vi "Read Cal Coefficients File.vi"() -> (0 "Original Coefficients":T1[](array[typedef]) {"Elapsed Time" format="%<%H:%M:%S>t"; "zero_utc" format="%x"; "cal_utc" format="%x"; "Pump Flow Rate" format="%0d"; "Number of Zeroes" format="%0d"; "V2C" format="%0d"; "C2V" format="%0d"; "duration" format="%<%H:%M:%S>t"; "DAC" format="%03x"; "mI" format="%.3g"; "V_(RA,15mA)" format="%0.4f"; "V_(RA,5mA)" format="%0.4f"; "Chamber Temp" format="%.1f"; "Humidity" format="%.1f"}, 1 "DATE":string, 2 "TYPE":string, 3 "CalFile Selected":path, 4 "PCB":string, 5 "Error":bool)   [LabVIEW 2016]
uses:
  Controls/Calibration Coefficients.ctl
  <vilib>/regexp/Match Regular Expression.xnode
panel:
  out "Lowc2v index":i32
  out "LowC2V":sgl[][](array[numeric]) format="%.3g"
  out "Lowc2v:size":i32
  out "End":bool
  out "Channel":string
  out "v2c index":i32
  out "c2v index":u8
  out "Char_current":sgl
  out "v2c:size":i32
  out "c2v:size":i32
  out "V2C":sgl[][](array[numeric]) format="%.3g"
  out "Spreadsheet":string[][](array[string])
  out "C2V":sgl[][](array[numeric]) format="%.3g"
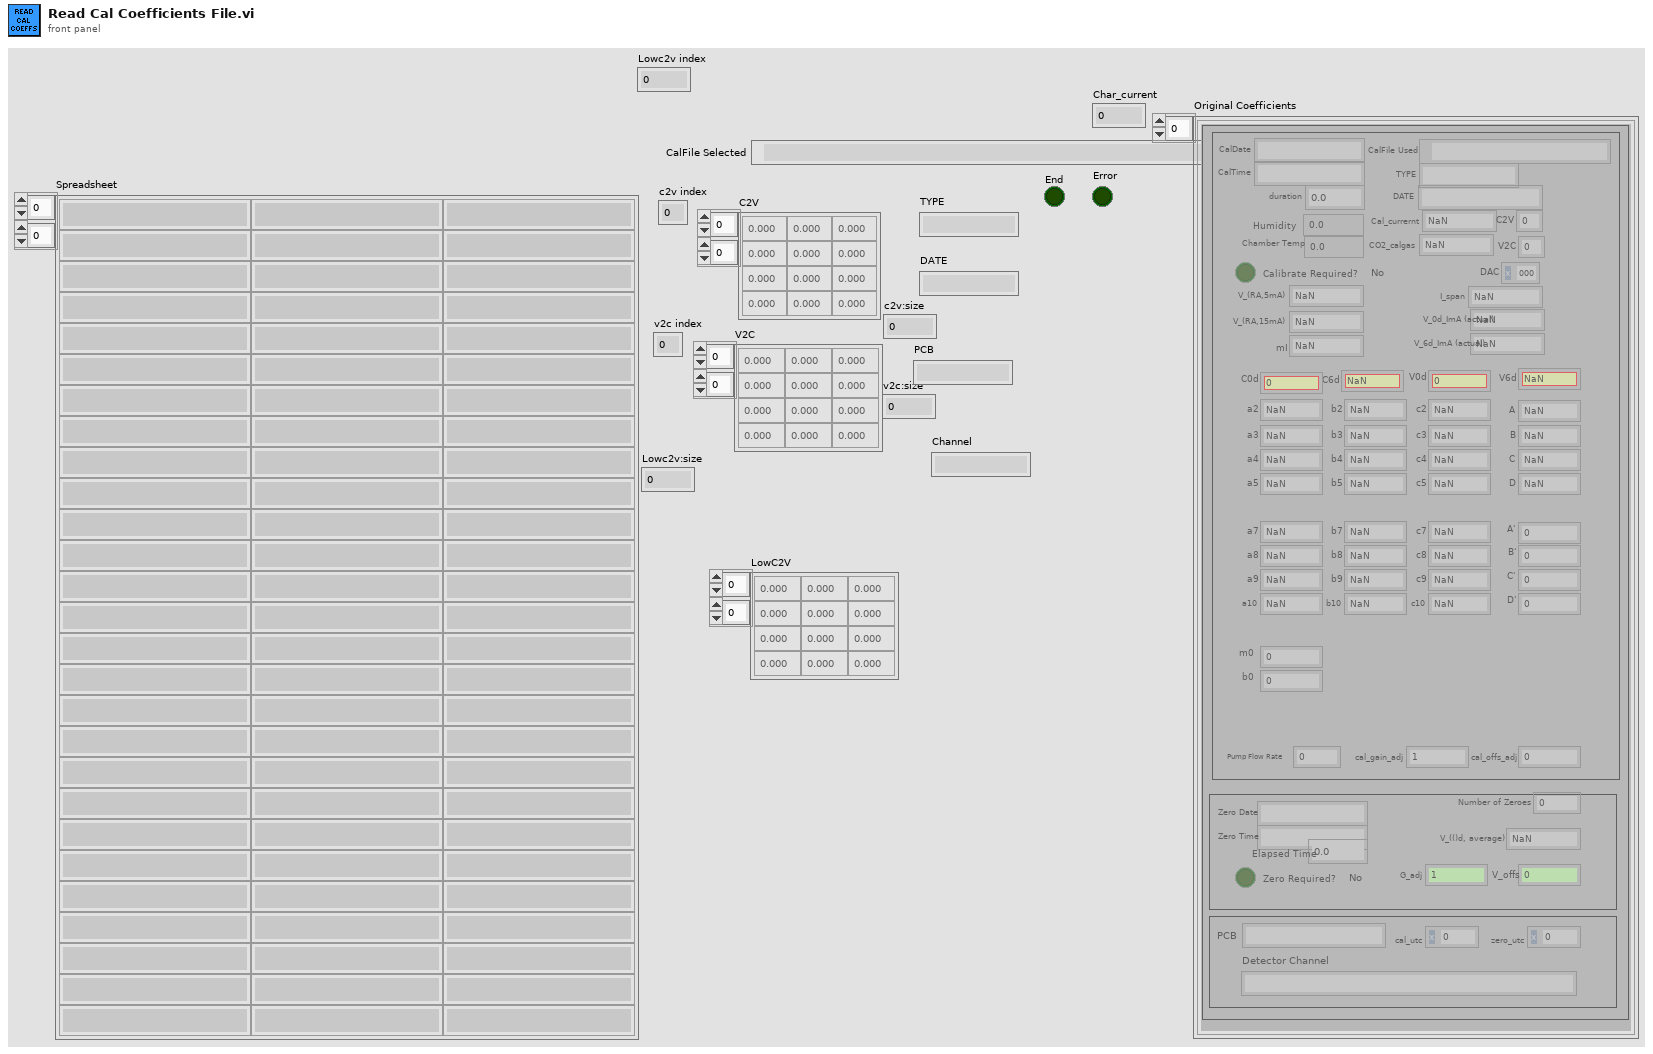
[diagram p1: front panel]
types:
  T1 = typedef "Calibration Coefficients.ctl" = cluster{"CalFile Used":path, "TYPE":string, "DATE":string, "Humidity":sgl, "Chamber Temp":dbl, "CO2_calgas":dbl, "V_(RA,5mA)":dbl, "V_(RA,15mA)":dbl, "mI":dbl, "V_0d_ImA (actual)":dbl, "V_6d_ImA (actual)":dbl, "I_span":dbl, "DAC":u16, "A":dbl, "B":dbl, "C":dbl, "D":dbl, "V6d":dbl, "A'":dbl, "B'":dbl, "C'":dbl, "D'":dbl, "V0d":dbl, "CalDate":string, "CalTime":string, "duration":dbl, "Detector Channel":string, "a2":dbl, "a3":dbl, "a4":dbl, "a5":dbl, "b2":dbl, "c2":dbl, "b3":dbl, "c3":dbl, "b4":dbl, "c4":dbl, "b5":dbl, "c5":dbl, "a7":dbl, "a8":dbl, "a9":dbl, "a10":dbl, "b7":dbl, "b8":dbl, "b9":dbl, "b10":dbl, "c7":dbl, "c8":dbl, "c9":dbl, "c10":dbl, "cal_offs_adj":dbl, "cal_gain_adj":dbl, "C6d":dbl, "C0d":dbl, "Cal_currernt":dbl, "C2V":u16, "V2C":u16, "Zero Date":string, "Zero Time":string, "Number of Zeroes":u16, "V_(()d, average)":dbl, "V_offs ":dbl, "G_adj":dbl, "Pump Flow Rate":u16, "Zero Required? ":bool, "Calibrate Required?":bool, "cal_utc":dbl, "zero_utc":dbl, "Elapsed Time":dbl, "PCB":string, "m0":dbl, "b0":dbl}
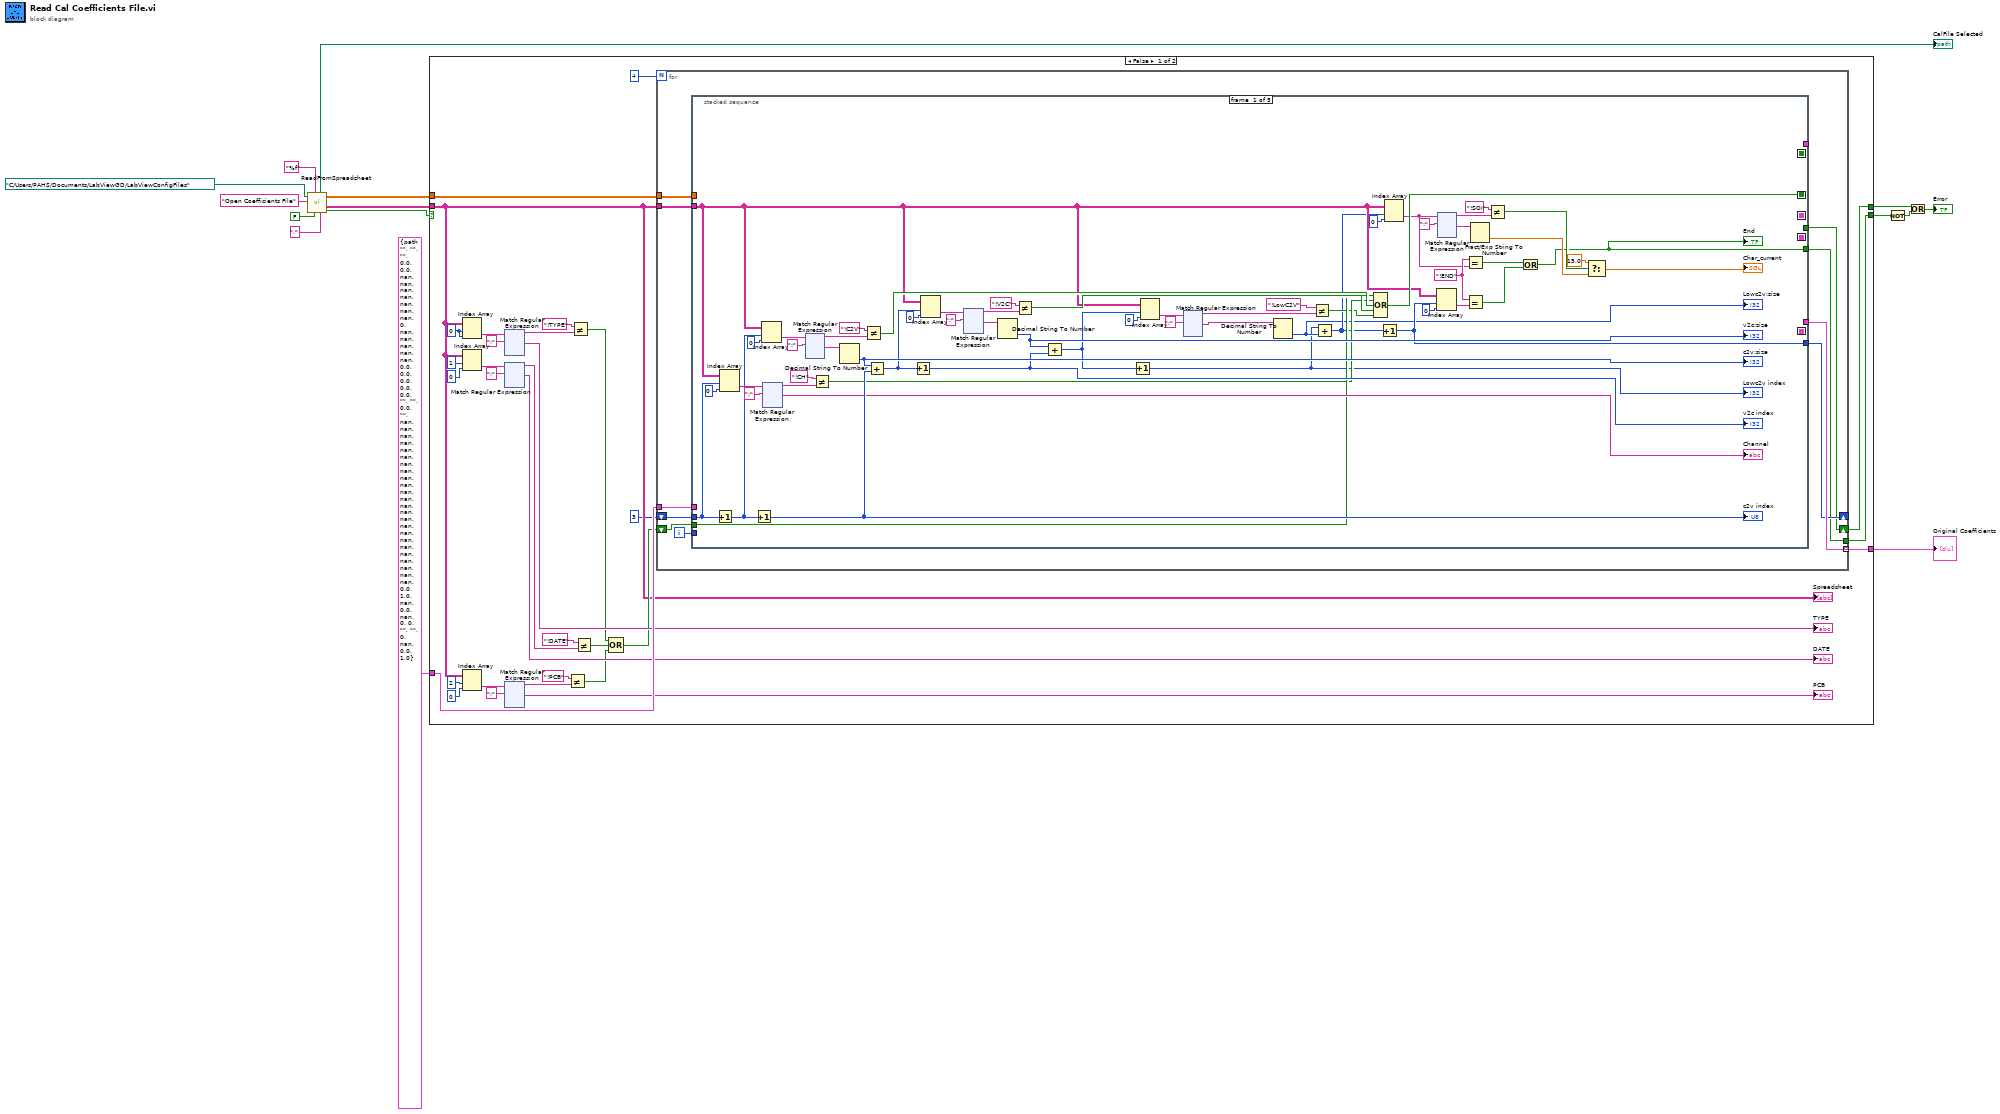
[diagram p0: block diagram]
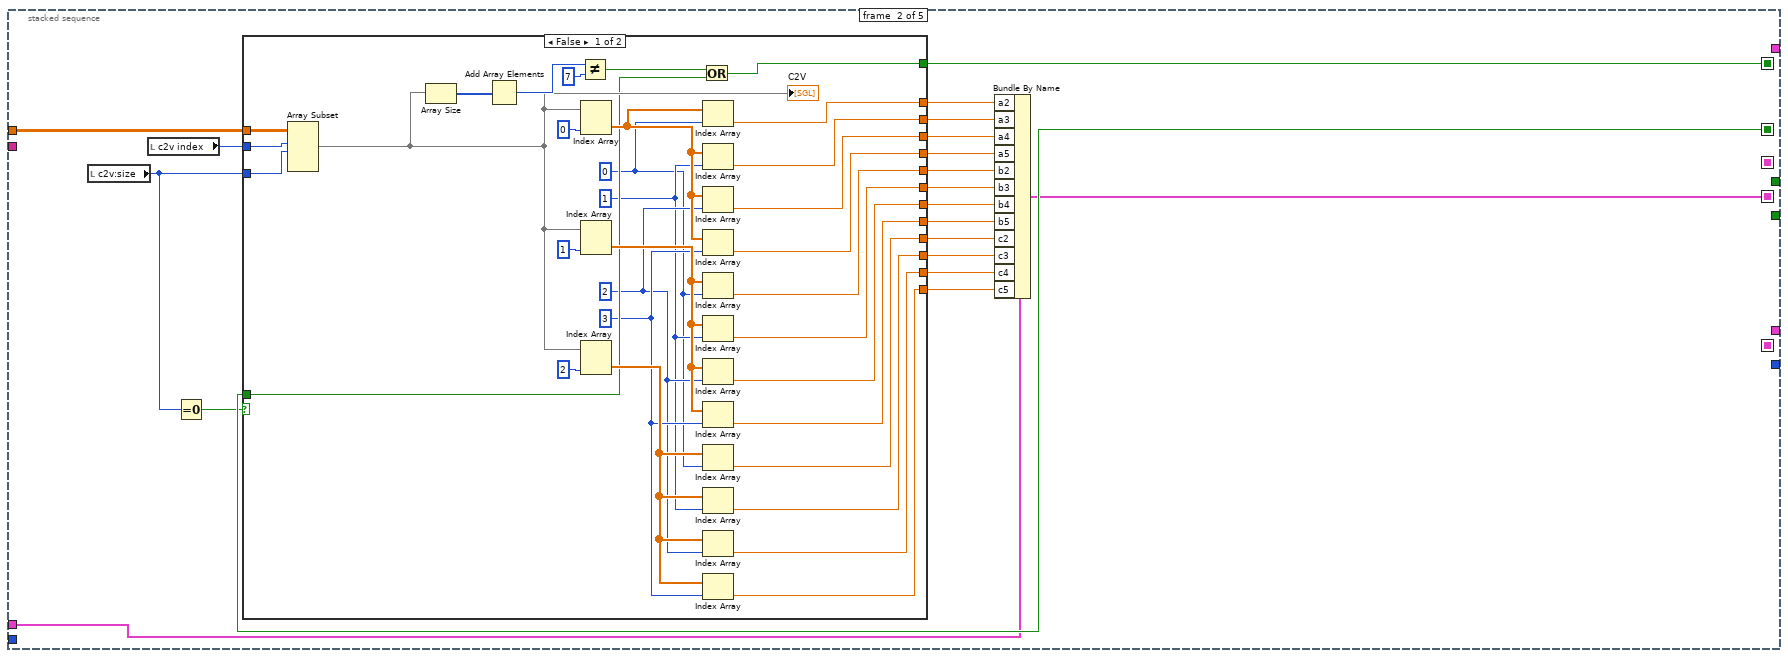
[diagram p2: hidden frame]
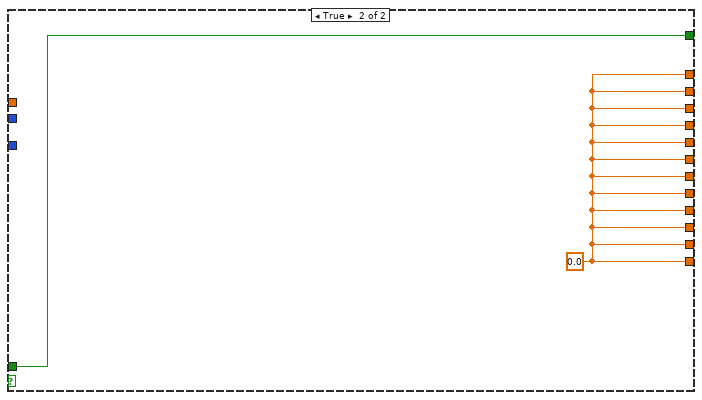
[diagram p3: hidden frame]
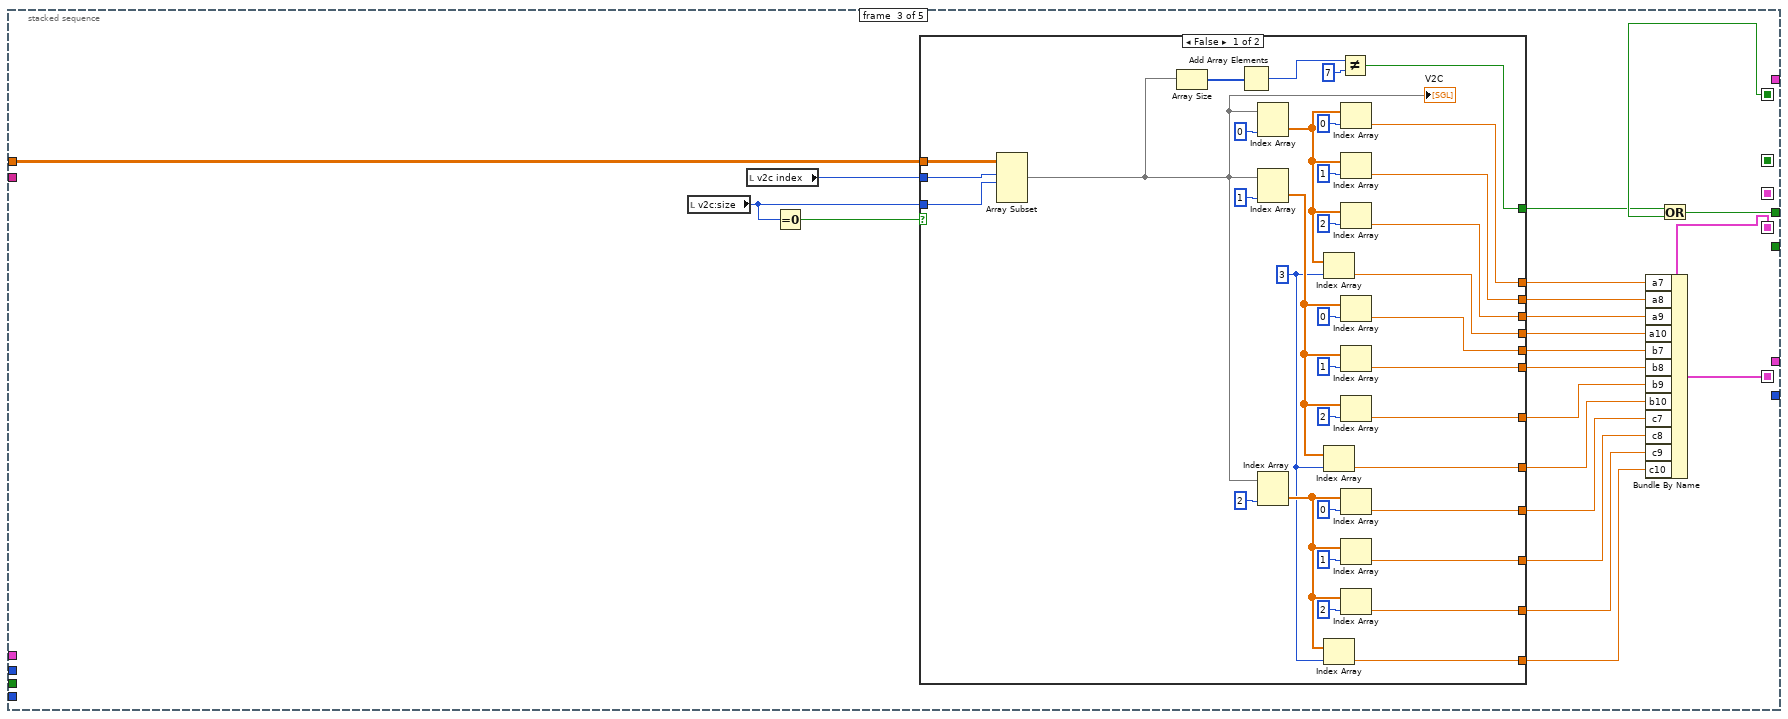
[diagram p4: hidden frame]
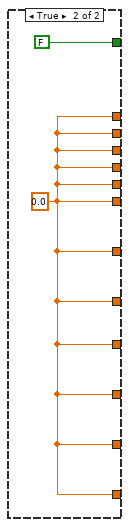
[diagram p5: hidden frame]
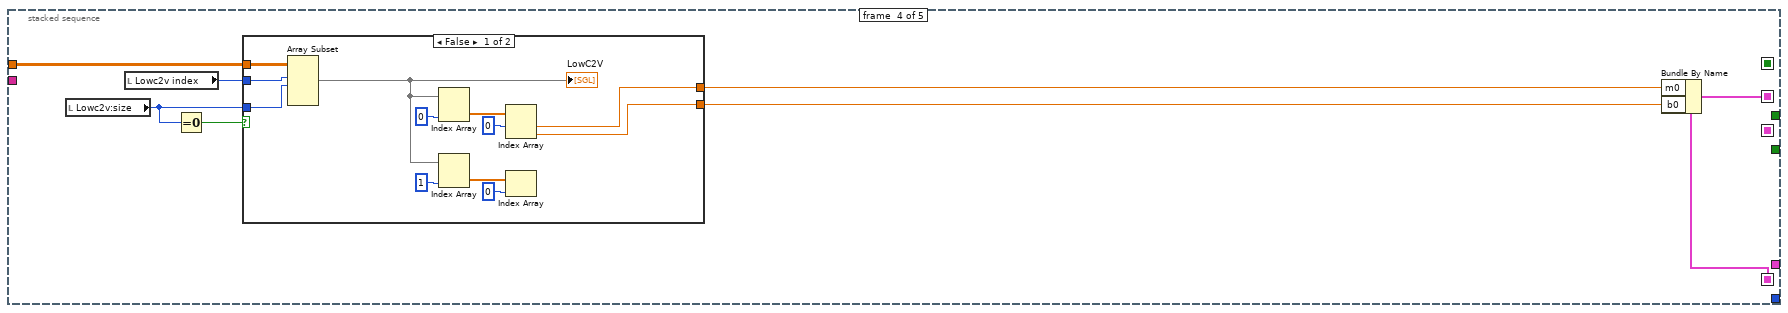
[diagram p6: hidden frame]
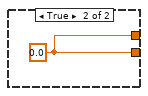
[diagram p7: hidden frame]
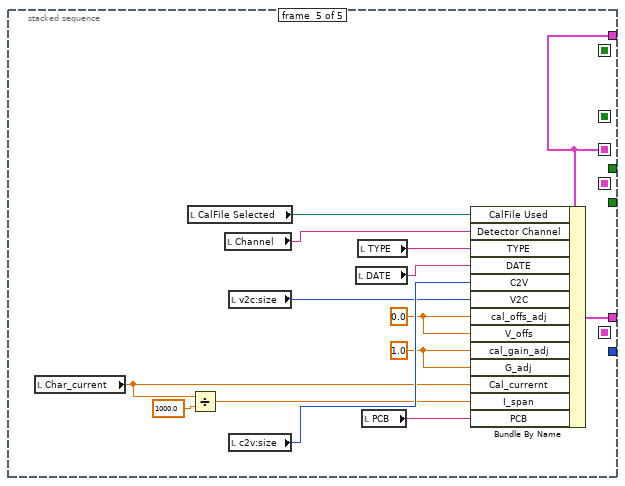
[diagram p8: hidden frame]
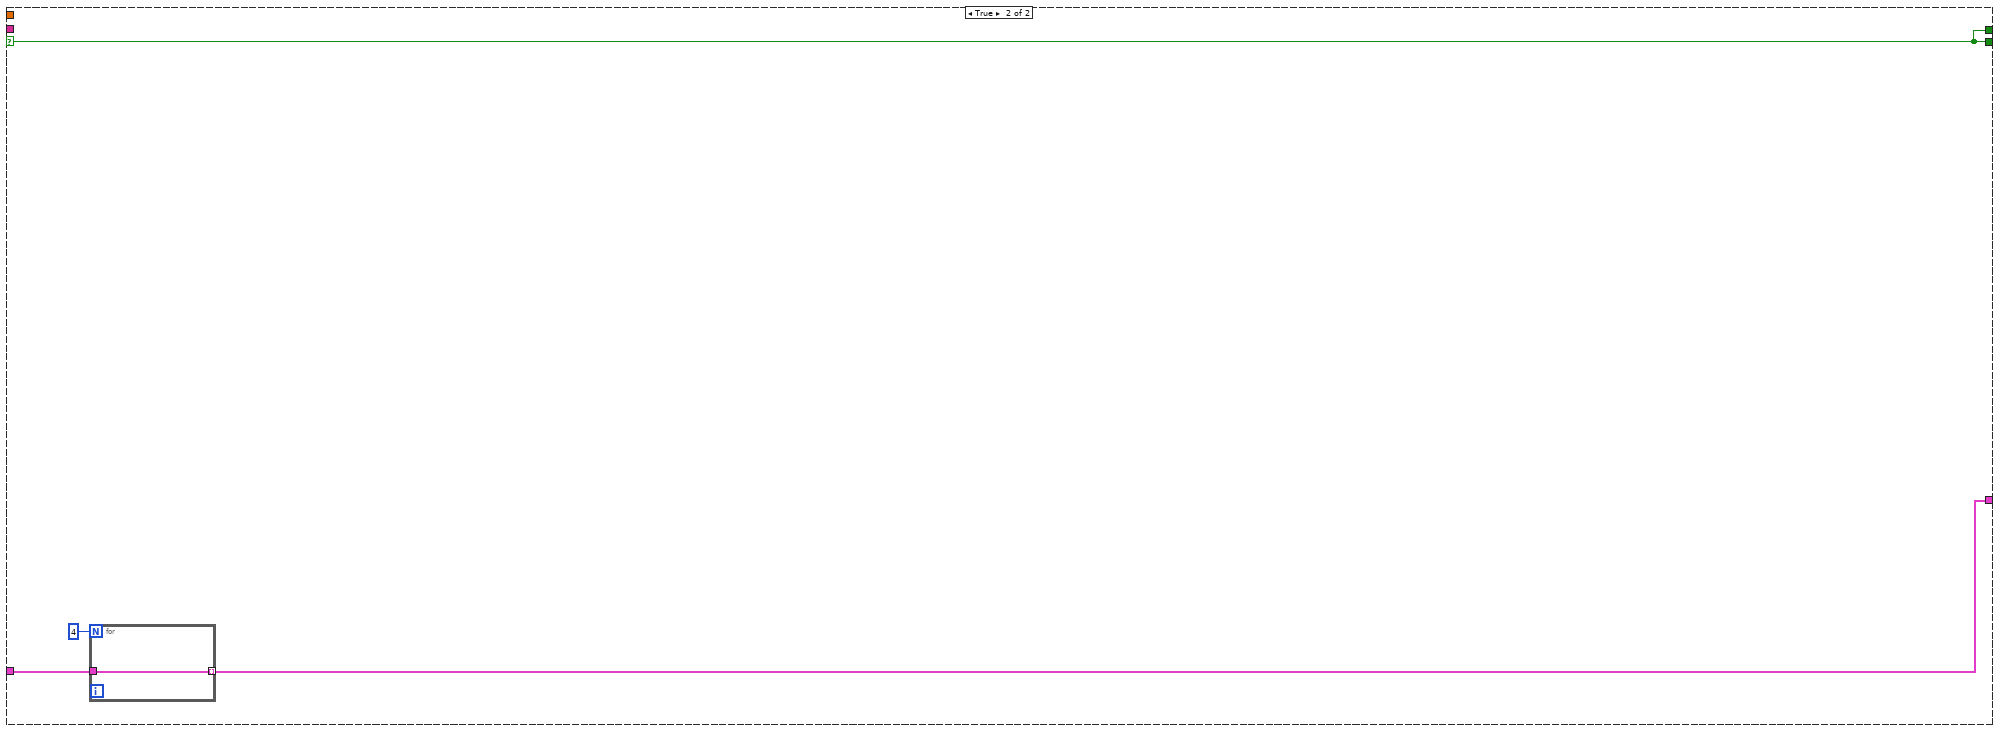
[diagram p9: hidden frame]
diagram:
  n1 = call "ReadFromSpreadsheet.vi"("delimiter (\\t)"="," ("delimiter (\\t)"), "transpose (no:F)"=FALSE, "format (%d)"="%f", "File Prompt"="Open Coefficients File", "file path"=path "C:/Users/PAHS/Documents/LabViewGD/LabViewConfigFiles") -> ("cancelled"=w9:bool, "text array"=w11:string[][], "all rows"=w10:sgl[][], "File Selected"=→"CalFile Selected":path)  [unwired: 2 in, 1 out]
  n2 = case shown="False" w9 {
    selector: w9 -> [_ w1177]
    tunnel: w11 -> [w18 _]
    tunnel: w10 -> [w47 _]
    tunnel: [w27 w1177] -> w4
    tunnel: T1 {"CalFile Used"=path "", "TYPE"="", "DATE"="", "Humidity"=0.0, "Chamber Temp"=0.0, "CO2_calgas"=nan, "V_(RA,5mA)"=nan, "V_(RA,15mA)"=nan, "mI"=nan, "V_0d_ImA (actual)"=nan, "V_6d_ImA (actual)"=nan, "I_span"=nan, "DAC"=0, "A"=nan, "B"=nan, "C"=nan, "D"=nan, "V6d"=nan, "A'"=0.0, "B'"=0.0, "C'"=0.0, "D'"=0.0, "V0d"=0.0, "CalDate"="", "CalTime"="", "duration"=0.0, "Detector Channel"="", "a2"=nan, "a3"=nan, "a4"=nan, "a5"=nan, "b2"=nan, "c2"=nan, "b3"=nan, "c3"=nan, "b4"=nan, "c4"=nan, "b5"=nan, "c5"=nan, "a7"=nan, "a8"=nan, "a9"=nan, "a10"=nan, "b7"=nan, "b8"=nan, "b9"=nan, "b10"=nan, "c7"=nan, "c8"=nan, "c9"=nan, "c10"=nan, "cal_offs_adj"=0.0, "cal_gain_adj"=1.0, "C6d"=nan, "C0d"=0.0, "Cal_currernt"=nan, "C2V"=0, "V2C"=0, "Zero Date"="", "Zero Time"="", "Number of Zeroes"=0, "V_(()d, average)"=nan, "V_offs "=0.0, "G_adj"=1.0, "Pump Flow Rate"=0, "Zero Required? "=FALSE, "Calibrate Required?"=FALSE, "cal_utc"=0.0, "zero_utc"=0.0, "Elapsed Time"=0.0, "PCB"="", "m0"=0.0, "b0"=0.0} ("Calibration Coefficients") -> [w46 w1180]
    tunnel: [w45 w1179] -> w7
    tunnel: [w26 w1177] -> w6
    frame False {
      w38 = 0
      n3 = Index Array(array=w18, index (row)=w38, index (col)=w38) -> (element=w39:string)
      n4 = Index Array(array=w18, index (row)=1, index (col)=0) -> (element=w42:string)
      n5 = Index Array(array=w18, index (row)=2, index (col)=0) -> (element=w21:string)
      n6 = xnode "Match Regular Expression"("input string"=w39, "regular expression"=":") -> ("before match"=w36:string, "after match"=→"TYPE":string)  [unwired: 4 in, 3 out]
      n7 = xnode "Match Regular Expression"("input string"=w42, "regular expression"=":") -> ("before match"=w34:string, "after match"=→"DATE":string)  [unwired: 4 in, 3 out]
      n8 = xnode "Match Regular Expression"("input string"=w21, "regular expression"=":") -> ("before match"=w23:string, "after match"=→"PCB":string)  [unwired: 4 in, 3 out]
      n9 = Not Equal?(x="!PCB", y=w23) -> (x != y?=w17:bool)
      n10 = Not Equal?(x="!TYPE", y=w36) -> (x != y?=w29:bool)
      n11 = Not Equal?(x="!DATE", y=w34) -> (x != y?=w30:bool)
      n12 = Compound Arithmetic op=OR(w29, w30, w17) -> (w28:bool)
      n13 = for {
        N: 4 -> [_]
        tunnel: w47 -> [w171]
        tunnel: w18 -> [w168]
        shift-right: [w165] -> _
        shift-left: 3 -> [w167]
        tunnel: w46 -> [w170]
        tunnel: [w169] -> w45 mode=indexing
        shift-right: [w163] -> w27
        shift-left: w28 -> [w164]
        tunnel: [w162] -> w26
        i -> [w166]
        n14 = stacked-sequence {
          seq-local: [w226 _ _ _ _] -> [_ w819 _ _ _]
          seq-local: [_ w815 _ _ _] -> [_ _ w862 _ _]
          seq-local: [_ w816 _ _ _] -> [_ _ w859 _ _]
          seq-local: [_ _ w861 _ _] -> [_ _ _ w915 _]
          seq-local: [_ _ _ w914 _] -> [_ _ _ _ w935]
          tunnel: w168 -> [w177 _ _ _ _]
          tunnel: w171 -> [_ w820 w875 w921 _]
          tunnel: w170 -> [_ w814 _ _ _]
          tunnel: [_ _ _ _ w946] -> w169
          tunnel: w167 -> [w216 _ _ _ _]
          tunnel: w166 -> [_ _ _ _ _]
          tunnel: [w184 _ _ _ _] -> w165
          tunnel: w164 -> [w186 _ _ _ _]
          tunnel: [_ _ w860 _ _] -> w163
          tunnel: [w188 _ _ _ _] -> w162
          tunnel: [_ _ _ _ w935] -> _
          frame #0 {
            w197 = "!END" ("x")
            n15 = Increment(x=w216) -> (x+1=w213:i32)
            n16 = Index Array(array=w177, index (row)=w216, index (col)=0) -> (element=w217:string)
            n17 = Increment(x=w213) -> (x+1=w212:i32)
            "c2v index" <- w212
            n18 = Index Array(array=w177, index (row)=w213, index (col)=0) -> (element=w224:string)
            n19 = xnode "Match Regular Expression"("input string"=w217, "regular expression"=":") -> ("before match"=w203:string, "after match"=→"Channel":string)  [unwired: 4 in, 3 out]
            n20 = xnode "Match Regular Expression"("input string"=w224, "regular expression"=":") -> ("before match"=w202:string, "after match"=w222:string)  [unwired: 4 in, 3 out]
            n21 = Not Equal?(x="!CH", y=w203) -> (x != y?=w185:bool)
            n22 = Decimal String To Number(string=w222) -> (number=w214:i32)  [unwired: 2 in, 1 out]
            "c2v:size" <- w214
            n23 = Not Equal?(x="!C2V", y=w202) -> (x != y?=w194:bool)
            n24 = Add(x=w214, y=w212) -> (x+y=w210:i32)
            n25 = Increment(x=w210) -> (x+1=w209:i32)
            "v2c index" <- w209
            n26 = Index Array(array=w177, index (row)=w210, index (col)=0) -> (element=w229:string)
            n27 = xnode "Match Regular Expression"("input string"=w229, "regular expression"=":") -> ("before match"=w192:string, "after match"=w227:string)  [unwired: 4 in, 3 out]
            n28 = Decimal String To Number(string=w227) -> (number=w211:i32)  [unwired: 2 in, 1 out]
            "v2c:size" <- w211
            n29 = Not Equal?(x="!V2C", y=w192) -> (x != y?=w193:bool)
            n30 = Add(x=w211, y=w209) -> (x+y=w175:i32)
            n31 = Increment(x=w175) -> (x+1=w172:i32)
            "Lowc2v index" <- w172
            n32 = Index Array(array=w177, index (row)=w175, index (col)=0) -> (element=w182:string)
            n33 = xnode "Match Regular Expression"("input string"=w182, "regular expression"=":") -> ("before match"=w179:string, "after match"=w180:string)  [unwired: 4 in, 3 out]
            n34 = Decimal String To Number(string=w180) -> (number=w173:i32)  [unwired: 2 in, 1 out]
            "Lowc2v:size" <- w173
            n35 = Not Equal?(x="!LowC2V", y=w179) -> (x != y?=w176:bool)
            n36 = Add(x=w172, y=w173) -> (x+y=w174:i32)
            n37 = Compound Arithmetic op=OR(w186, w185, w194, w193, w176) -> (w226:bool)
            n38 = Increment(x=w174) -> (x+1=w184:i32)
            n39 = Index Array(array=w177, index (row)=w174, index (col)=0) -> (element=w189:string)
            n40 = Index Array(array=w177, index (row)=w184, index (col)=0) -> (element=w190:string)
            n41 = xnode "Match Regular Expression"("input string"=w189, "regular expression"=":") -> ("before match"=w198:string, "after match"=w219:string)  [unwired: 4 in, 3 out]
            n42 = Equal?(x=w197, y=w189) -> (x = y?=w195:bool)
            n43 = Equal?(x=w197, y=w190) -> (x = y?=w196:bool)
            n44 = Fract/Exp String To Number(string=w219) -> (number=w207:dbl)  [unwired: 3 in, 1 out]
            n45 = Not Equal?(x="!SOI", y=w198) -> (x != y?=w191:bool)
            n46 = Or(x=w195, y=w196) -> (x .or. y?=w188:bool)
            "End" <- w188
            n47 = Select(t=15.0, s=w191, f=w207) -> (s? t:f=→"Char_current":dbl)
          }
          frame #1 {
            n48 = local read "c2v:size"() -> (w801:i32)
            n49 = local read "c2v index"() -> (w817:u8)
            n50 = Equal To 0?(x=w801) -> (x = 0?=w818:bool)
            n51 = case shown="False" w818 {
              tunnel: w820 -> [w852 _]
              tunnel: w819 -> [w840 w854]
              tunnel: w817 -> [w834 _]
              tunnel: [w839 w854] -> w816
              tunnel: [w833 w853] -> w813
              tunnel: [w832 w853] -> w812
              tunnel: [w831 w853] -> w811
              tunnel: [w830 w853] -> w810
              tunnel: [w829 w853] -> w809
              tunnel: [w828 w853] -> w808
              tunnel: [w827 w853] -> w807
              tunnel: [w826 w853] -> w806
              tunnel: [w825 w853] -> w805
              tunnel: [w824 w853] -> w804
              tunnel: [w823 w853] -> w803
              tunnel: [w822 w853] -> w802
              tunnel: w801 -> [w821 _]
              frame False {
                w838 = 3 ("index")
                w837 = 2 ("index")
                w836 = 1 ("index")
                w835 = 0 ("index")
                n52 = Array Subset(array=w852, index (row)=w834, length (row)=w821) -> (w842:sgl[][])  [unwired: 2 in]
                "C2V" <- w842
                n53 = Array Size(array=w842) -> (size(s)=w851:i32[])
                n54 = Add Array Elements(numeric array=w851) -> (sum=w850:i32)
                n55 = Not Equal?(x=w850, y=7) -> (x != y?=w841:bool)
                n56 = Index Array(array=w842, index (col)=0 ("disabled index (col)")) -> (element=w847:sgl[])  [unwired: 1 in]
                n57 = Index Array(array=w842, index (col)=1 ("disabled index (col)")) -> (element=w844:sgl[])  [unwired: 1 in]
                n58 = Index Array(array=w842, index (col)=2 ("disabled index (col)")) -> (element=w843:sgl[])  [unwired: 1 in]
                n59 = Or(x=w841, y=w840) -> (x .or. y?=w839:bool)
                n60 = Index Array(array=w847, index=w835) -> (element=w833:sgl)
                n61 = Index Array(array=w847, index=w836) -> (element=w832:sgl)
                n62 = Index Array(array=w847, index=w837) -> (element=w831:sgl)
                n63 = Index Array(array=w847, index=w838) -> (element=w822:sgl)
                n64 = Index Array(array=w844, index=w835) -> (element=w830:sgl)
                n65 = Index Array(array=w844, index=w836) -> (element=w829:sgl)
                n66 = Index Array(array=w844, index=w837) -> (element=w828:sgl)
                n67 = Index Array(array=w844, index=w838) -> (element=w827:sgl)
                n68 = Index Array(array=w843, index=w835) -> (element=w826:sgl)
                n69 = Index Array(array=w843, index=w836) -> (element=w825:sgl)
                n70 = Index Array(array=w843, index=w837) -> (element=w824:sgl)
                n71 = Index Array(array=w843, index=w838) -> (element=w823:sgl)
              }
              frame True {
                w853 = sgl 0.0
              }
            }
            n72 = Bundle By Name(cluster=w814, "a2"=w813, "a3"=w812, "a4"=w811, "a5"=w802, "b2"=w810, "b3"=w809, "b4"=w808, "b5"=w807, "c2"=w806, "c3"=w805, "c4"=w804, "c5"=w803) -> (w815:T1)
          }
          frame #2 {
            n73 = local read "v2c:size"() -> (w855:i32)
            n74 = local read "v2c index"() -> (w856:i32)
            n75 = Equal To 0?(x=w855) -> (x = 0?=w857:bool)
            n76 = case shown="False" w857 {
              tunnel: w875 -> [w911 _]
              tunnel: [w906 w912] -> w874
              tunnel: [w905 w912] -> w873
              tunnel: [w904 w912] -> w872
              tunnel: [w902 w912] -> w871
              tunnel: [w888 w912] -> w870
              tunnel: [w887 w912] -> w869
              tunnel: [w886 w912] -> w868
              tunnel: [w885 w912] -> w867
              tunnel: [w884 w912] -> w866
              tunnel: [w883 w912] -> w865
              tunnel: [w882 w912] -> w864
              tunnel: [w881 w912] -> w863
              tunnel: w856 -> [w878 _]
              tunnel: [w877 FALSE] -> w858
              tunnel: w855 -> [w876 _]
              frame False {
                w879 = 3 ("index")
                n77 = Array Subset(array=w911, index (row)=w878, length (row)=w876) -> (w880:sgl[][])  [unwired: 2 in]
                "V2C" <- w880
                n78 = Array Size(array=w880) -> (size(s)=w910:i32[])
                n79 = Add Array Elements(numeric array=w910) -> (sum=w909:i32)
                n80 = Index Array(array=w880, index (col)=0 ("disabled index (col)")) -> (element=w903:sgl[])  [unwired: 1 in]
                n81 = Index Array(array=w880, index (col)=1 ("disabled index (col)")) -> (element=w890:sgl[])  [unwired: 1 in]
                n82 = Index Array(array=w880, index (col)=2 ("disabled index (col)")) -> (element=w889:sgl[])  [unwired: 1 in]
                n83 = Index Array(array=w903, index=w879) -> (element=w902:sgl)
                n84 = Index Array(array=w890, index=w879) -> (element=w885:sgl)
                n85 = Index Array(array=w889, index=w879) -> (element=w881:sgl)
                n86 = Not Equal?(x=w909, y=7) -> (x != y?=w877:bool)
                n87 = Index Array(array=w903, index=0) -> (element=w906:sgl)
                n88 = Index Array(array=w903, index=1) -> (element=w905:sgl)
                n89 = Index Array(array=w903, index=2) -> (element=w904:sgl)
                n90 = Index Array(array=w890, index=0) -> (element=w888:sgl)
                n91 = Index Array(array=w890, index=1) -> (element=w887:sgl)
                n92 = Index Array(array=w890, index=2) -> (element=w886:sgl)
                n93 = Index Array(array=w889, index=0) -> (element=w884:sgl)
                n94 = Index Array(array=w889, index=1) -> (element=w883:sgl)
                n95 = Index Array(array=w889, index=2) -> (element=w882:sgl)
              }
              frame True {
                w912 = sgl 0.0
              }
            }
            n96 = Bundle By Name(cluster=w862, "a7"=w874, "a8"=w873, "a9"=w872, "a10"=w871, "b7"=w870, "b8"=w869, "b9"=w868, "b10"=w867, "c7"=w866, "c8"=w865, "c9"=w864, "c10"=w863) -> (w861:T1)
            n97 = Or(x=w858, y=w859) -> (x .or. y?=w860:bool)
          }
          frame #3 {
            n98 = local read "Lowc2v:size"() -> (w918:i32)
            n99 = local read "Lowc2v index"() -> (w919:i32)
            n100 = Equal To 0?(x=w918) -> (x = 0?=w920:bool)
            n101 = case shown="False" w920 {
              tunnel: w921 -> [w933 _]
              tunnel: [w931 w934] -> w917
              tunnel: [w922 w934] -> w916
              tunnel: w919 -> [w924 _]
              tunnel: w918 -> [w923 _]
              frame False {
                n102 = Array Subset(array=w933, index (row)=w924, length (row)=w923) -> (w925:sgl[][])  [unwired: 2 in]
                "LowC2V" <- w925
                n103 = Index Array(array=w925, index (col)=0 ("disabled index (col)")) -> (element=w930:sgl[])  [unwired: 1 in]
                n104 = Index Array(array=w925, index (col)=1 ("disabled index (col)")) -> (element=w926:sgl[])  [unwired: 1 in]
                n105 = Index Array(array=w930, index #1=0 ("index")) -> (element #1=w931:sgl, element #2=w922:sgl)  [unwired: 1 in]
                n106 = Index Array(array=w926, index=0) -> ()  [unwired: 1 out]
              }
              frame True {
                w934 = sgl 0.0
              }
            }
            n107 = Bundle By Name(cluster=w915, "m0"=w917, "b0"=w916) -> (w914:T1)
          }
          frame #4 {
            w942 = 1.0
            w943 = 0.0
            n108 = local read "Char_current"() -> (w939:sgl)
            n109 = local read "CalFile Selected"() -> (w938:path)
            n110 = Divide(x=w939, y=sgl 1000.0) -> (x/y=w940:sgl)
            n111 = local read "Channel"() -> (w937:string)
            n112 = local read "v2c:size"() -> (w944:i32)
            n113 = local read "c2v:size"() -> (w945:i32)
            n114 = local read "DATE"() -> (w948:string)
            n115 = local read "TYPE"() -> (w947:string)
            n116 = local read "PCB"() -> (w936:string)
            n117 = Bundle By Name(cluster=w935, "CalFile Used"=w938, "Detector Channel"=w937, "TYPE"=w947, "DATE"=w948, "C2V"=w945, "V2C"=w944, "cal_offs_adj"=w943, "V_offs"=w943, "cal_gain_adj"=w942, "G_adj"=w942, "Cal_currernt"=w939, "I_span"=w940, "PCB"=w936) -> (w946:T1)
          }
        }
      }
      "Spreadsheet" <- w18
    }
    frame True {
      n118 = for {
        N: 4 -> [_]
        tunnel: w1180 -> [w1181]
        tunnel: [w1181] -> w1179 mode=indexing
      }
    }
  }
  "Original Coefficients" <- w7
  n119 = Not(x=w6) -> (.not. x?=w5:bool)
  n120 = Or(x=w4, y=w5) -> (x .or. y?=→"Error":bool)
